vi "Write Encoder Converter.vi"(10 "Enccoder Converter":T1 {"Distance Per Count" format="%.3f"}, 11 "EncoderConverter in":refnum<class "EncoderConverter.lvclass">) -> (3 "EncoderConverter out":refnum<class "EncoderConverter.lvclass">)   [LabVIEW 2013, in "EncoderConverter.lvlib" / "EncoderConverter.lvclass"]
uses:
  <userlib>/Common/Devices/EncoderConverter/EncoderConverter/EncoderConverter.lvclass
  <userlib>/Common/Devices/EncoderConverter/Config/EncoderConverter.ctl
  <userlib>/Common/Devices/EncoderConverter/EncoderConverter/EncoderConverter.lvclass/EncoderConverter.ctl
  <userlib>/Common/Devices/EncoderConverter/EncoderConverter.lvlib
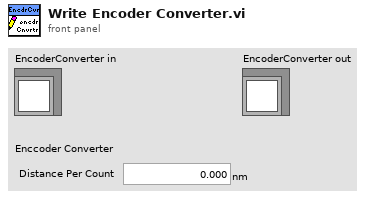
[diagram p1: front panel]
types:
  T1 = typedef "EncoderConverter.lvlib/EncoderConverter.ctl" = cluster{"Distance Per Count":dbl[unit]}
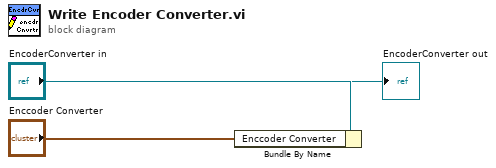
[diagram p0: block diagram]
diagram:
  n1 = Bundle By Name(cluster="EncoderConverter in", "Enccoder Converter"="Enccoder Converter") -> (→"EncoderConverter out":refnum<class "EncoderConverter.lvclass">)
